vi "Initialize Object Map.vi"(8 "error in":errorcluster, 9 "object name":string, 10 "status channel map":map{string, map{string, i32}}(c390), 11 "object map in":T1) -> (0 "error out":errorcluster, 3 "object map out":T1)   [LabVIEW 2019, in "HLA Custom Device Engine.lvlib"]
uses:
  HLA Custom Device Engine.lvlib
  _typedefs/map_object_value.ctl
  _typedefs/map_attr_param_data.ctl
  emea-ni-adg-hla-lv/src/helpers/Attribute Handle Set/ahs.lvlib
  emea-ni-adg-hla-lv/src/helpers/Attribute Handle Value Map/ahvm.lvlib
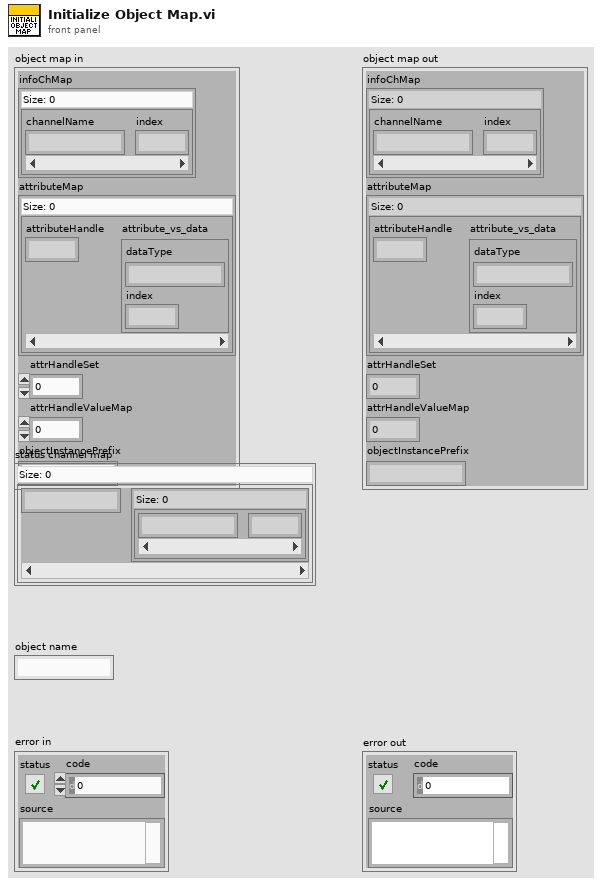
[diagram p1: front panel]
types:
  T1 = typedef "HLA Custom Device Engine.lvlib/map_object_value.ctl" = cluster{"infoChMap":map{string, i32}, "attributeMap":map{u64, T2}, "attrHandleSet":u64, "attrHandleValueMap":u64, "objectInstancePrefix":string}
  T2 = typedef "HLA Custom Device Engine.lvlib/map_attr_param_data.ctl" = cluster{"dataType":string, "index":i32}
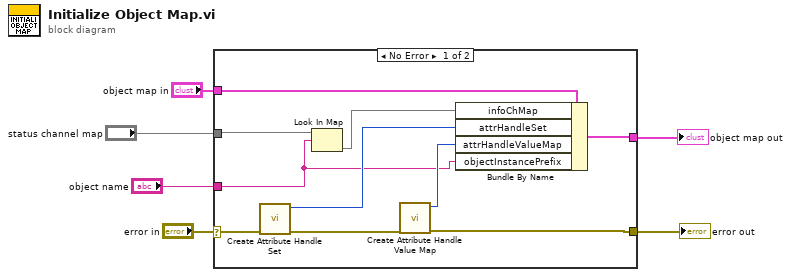
[diagram p0: block diagram]
diagram:
  n1 = case shown="No Error" "error in" {
    selector: "error in" -> [w12 w18]
    tunnel: "object name" -> [w7 _]
    tunnel: [w16 w17] -> w5
    tunnel: "object map in" -> [w14 w17]
    tunnel: "status channel map" -> [w13 _]
    tunnel: [w8 w18] -> w1
    frame No Error {
      n2 = call "Create Attribute Handle Set.vi"("error in"=w12) -> ("error out"=w10:errorcluster, "attrHandleSet"=w11:u64)  [unwired: 9 in]
      n3 = Look In Map(map=w13, key=w7) -> (value=w15:map{string, i32})  [unwired: 1 in, 1 out]
      n4 = call "Create Attribute Handle Value Map.vi"("error in"=w10) -> ("error out"=w8:errorcluster, "attrHandleValueMap"=w9:u64)  [unwired: 9 in]
      n5 = Bundle By Name(cluster=w14, "infoChMap"=w15, "attrHandleSet"=w11, "attrHandleValueMap"=w9, "objectInstancePrefix"=w7) -> (w16:T1)
    }
    frame Error {
    }
  }
  "object map out" <- w5
  "error out" <- w1
